vi "ListIDs.vi"(8 "Old IDs (optional)":u32[](array[numeric]), 11 "New IDs":u32[](array[numeric])) -> (3 "Buffer":u32[](array[numeric]))   [LabVIEW 2016, in "DSI-RT.lvlib"]
uses:
  DSI-RT.lvlib
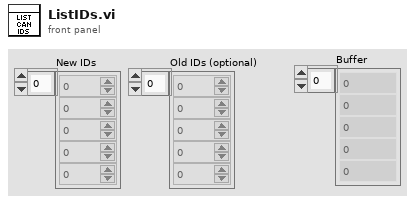
[diagram p1: front panel]
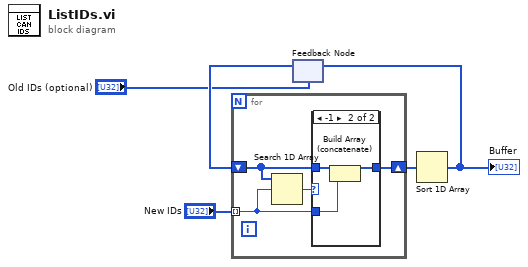
[diagram p0: block diagram]
diagram:
  n1 = feedback #1("Old IDs (optional)") -> (w2:u32[])
  n2 = for {
    tunnel: "New IDs" -> [w8] mode=indexing
    shift-right: [w7] -> w4
    shift-left: w2 -> [w6]
    n3 = Search 1D Array(1D array=w6, element=w8) -> (index of element=w9:i32)  [unwired: 1 in]
    n4 = case shown="-1" w9 {
      tunnel: w8 -> [_ w13]
      tunnel: [w10 w11] -> w7
      tunnel: w6 -> [w10 w12]
      frame Default {
      }
      frame -1 {
        n5 = Build Array (concatenate)(w12, w13) -> (w11:u32[])
      }
    }
  }
  n6 = Sort 1D Array(array=w4) -> (sorted array=w3:u32[])
  "Buffer" <- w3
  n7 = feedback-in #1(w3) -> ()
